vi "playback wrist.vi"(4 "Home":bool, 5 "Rewind":bool, 7 "Playback":bool, 8 "Taper Limit":dbl=1.0, 9 "Playback allow":bool=TRUE, 10 "Encoder Recording Data":cluster{dbl, u32}[](array[cluster])=[{0.0, 20}, {0.0, 41}, {0.0, 60}, {0.0, 80}, {0.0, 100}, {0.0, 120}, {0.0, 140}, {0.0, 160}, {0.0, 180}, {0.0, 200}, {0.0, 220}, {0.0, 245}, {0.0, 263}, {0.0, 284}, {0.0, 303}, {0.0, 325}, {0.0, 343}, {0.0, 364}, {0.0, 385}, {0.0, 406}, {0.0, 422}, {0.0, 442}, {0.0, 465}, {0.0, 486}, {0.0, 510}, {0.0, 527}, {0.0, 547}, {0.0, 567}, {0.0, 587}, {0.0, 606}, {0.0, 626}, {0.0, 649}, {0.0, 669}, {0.0, 689}, {0.0, 709}, {0.0, 730}, {0.0, 749}, {0.25, 769}, {0.75, 789}, {1.5, 809}, {2.75, 830}, {4.5, 849}, {7.25, 870}, {11.25, 891}, {16.25, 913}, {21.25, 931}, {28.5, 952}, {36.75, 974}, {45.75, 993}, {55.75, 1013}, {64.5, 1031}, {75.5, 1052}, {87.5, 1073}, {99.5, 1093}, {111.0, 1114}, {123.0, 1133}, {136.0, 1155}, {147.0, 1174}, {158.25, 1194}, {169.75, 1214}, {181.5, 1235}, {192.25, 1254}, {203.0, 1275}, {215.25, 1297}, {225.75, 1317}, {236.25, 1337}, {247.25, 1357}, {259.25, 1379}, {270.25, 1399}, {280.0, 1417}, {290.5, 1438}, {300.75, 1458}, {311.25, 1478}, {321.25, 1499}, {331.75, 1519}, {341.75, 1540}, {351.0, 1559}, {361.0, 1580}, {370.5, 1599}, {379.25, 1619}, {389.0, 1639}, {398.5, 1660}, {407.5, 1679}, {417.0, 1699}, {426.75, 1720}, {436.0, 1740}, {445.25, 1760}, {457.5, 1787}, {464.25, 1801}, {474.75, 1823}, {482.75, 1841}, {493.5, 1864}, {503.0, 1884}, {511.75, 1903}, {521.75, 1925}, {530.5, 1945}, {540.25, 1966}, {549.0, 1986}, {558.0, 2006}, {567.25, 2027}, {576.0, 2047}, {585.5, 2068}, {594.75, 2087}, {604.0, 2107}, {613.5, 2127}, {623.25, 2147}, {632.75, 2167}, {643.5, 2189}, {652.75, 2208}, {661.5, 2227}, {671.5, 2248}, {680.75, 2268}, {690.25, 2288}, {700.25, 2309}, {709.75, 2329}, {718.5, 2347}, {728.25, 2369}, {737.0, 2389}, {745.25, 2408}, {753.75, 2429}, {761.25, 2448}, {769.25, 2469}, {776.0, 2488}, {783.25, 2508}, {790.0, 2528}, {797.0, 2549}, {803.5, 2570}, {809.75, 2590}, {815.25, 2610}, {819.5, 2630}, {823.0, 2651}, {825.75, 2674}, {829.75, 2694}, {832.75, 2712}, {835.75, 2733}, {837.5, 2755}, {839.0, 2775}, {840.25, 2795}, {841.25, 2815}, {842.5, 2836}, {843.0, 2855}, {843.5, 2875}, {843.5, 2896}, {843.75, 2917}, {846.5, 2937}, {850.25, 2957}, {851.25, 2977}, {851.25, 2997}, {851.25, 3016}, {851.25, 3037}, {851.25, 3057}, {851.25, 3077}, {850.75, 3097}, {850.5, 3117}, {850.5, 3137}, {850.25, 3157}, {850.25, 3178}, {850.25, 3198}, {850.25, 3218}, {851.25, 3238}, {851.5, 3258}, {851.5, 3278}, {851.5, 3298}, {851.75, 3318}, {851.75, 3339}, {851.75, 3359}, {851.75, 3380}, {851.75, 3400}, {851.75, 3420}, {851.75, 3444}, {851.75, 3460}, {851.75, 3481}, {851.75, 3500}, {851.75, 3520}, {851.75, 3541}, {851.75, 3562}, {851.75, 3580}, {851.75, 3600}, {851.75, 3620}, {851.75, 3641}, {851.75, 3664}, {852.0, 3680}, {852.0, 3701}, {852.0, 3720}, {852.0, 3741}, {852.0, 3761}, {852.0, 3781}, {852.0, 3805}, {852.0, 3821}, {852.0, 3844}, {852.0, 3865}, {852.0, 3886}, {852.0, 3904}, {852.0, 3927}, {852.0, 3945}, {852.0, 3965}, {852.0, 3985}, {852.0, 4007}, {852.0, 4026}, {852.0, 4045}, {852.0, 4066}, {852.0, 4087}, {852.0, 4108}, {852.0, 4129}, {852.0, 4149}, {852.0, 4169}, {852.0, 4190}, {852.0, 4209}, {852.0, 4229}, {852.0, 4250}, {852.0, 4270}, {852.0, 4289}, {852.0, 4309}, {852.0, 4329}, {852.0, 4349}, {852.0, 4369}, {852.0, 4389}, {852.0, 4409}, {852.0, 4429}, {852.0, 4449}, {852.0, 4469}, {852.0, 4490}, {852.0, 4511}, {852.0, 4529}, {852.0, 4549}, {852.0, 4570}, {852.0, 4590}, {852.0, 4609}, {852.0, 4629}, {852.0, 4650}, {852.0, 4669}, {852.0, 4690}, {852.0, 4710}, {852.0, 4730}, {852.0, 4751}, {852.0, 4770}, {852.0, 4790}, {852.0, 4811}, {852.0, 4830}, {852.0, 4854}, {852.0, 4874}, {852.0, 4894}, {852.0, 4910}, {852.0, 4933}, {852.0, 4951}, {852.0, 4971}, {852.0, 4993}, {852.0, 5013}, {852.0, 5034}, {852.0, 5053}, {852.0, 5074}, {852.0, 5094}, {852.0, 5112}, {852.0, 5134}, {852.0, 5154}, {852.0, 5173}, {851.25, 5193}, {850.25, 5213}, {849.0, 5232}, {847.0, 5254}, {845.25, 5277}, {845.0, 5296}, {844.75, 5315}, {843.25, 5335}, {843.25, 5354}, {843.0, 5376}, {843.0, 5396}, {843.0, 5415}, {843.0, 5435}, {843.0, 5454}, {843.0, 5474}, {843.0, 5496}, {843.0, 5516}, {843.0, 5534}, {843.0, 5555}, {843.0, 5576}, {842.75, 5595}, {842.75, 5614}, {842.75, 5634}, {842.75, 5654}, {842.5, 5677}, {842.0, 5698}, {840.75, 5717}, {838.5, 5738}, {835.75, 5759}, {832.0, 5779}, {828.25, 5799}, {824.25, 5820}, {820.25, 5838}, {815.25, 5859}, {810.25, 5879}, {804.25, 5900}, {798.0, 5918}, {790.5, 5938}, {782.0, 5958}, {771.75, 5979}, {762.0, 5999}, {751.5, 6019}, {739.75, 6040}, {729.5, 6059}, {718.0, 6079}, {707.25, 6098}, {694.5, 6120}, {683.75, 6138}, {671.75, 6159}, {659.5, 6179}, {647.25, 6200}, {635.75, 6219}, {624.25, 6240}, {610.0, 6264}, {601.75, 6279}, {590.75, 6300}, {580.0, 6321}, {569.75, 6340}, {558.75, 6362}, {549.5, 6380}, {540.75, 6399}, {531.5, 6419}, {522.5, 6439}, {512.75, 6462}, {505.0, 6480}, {496.0, 6500}, {488.25, 6519}, {479.5, 6539}, {471.0, 6559}, {462.25, 6580}, {454.0, 6600}, {445.75, 6620}, {438.0, 6639}, {429.5, 6660}, {421.25, 6679}, {413.0, 6699}, {404.25, 6720}, {395.5, 6740}, {386.75, 6760}, {377.75, 6781}, {368.75, 6803}, {360.75, 6821}, {349.75, 6847}, {339.75, 6867}, {330.5, 6886}, {320.5, 6906}, {309.5, 6927}, {298.0, 6949}, {286.0, 6970}, {274.25, 6991}, {262.0, 7011}, {250.25, 7030}, {237.5, 7051}, {223.25, 7074}, {210.5, 7094}, {199.25, 7111}, {184.25, 7133}, {173.5, 7150}, {157.5, 7174}, {144.0, 7194}, {130.25, 7214}, {117.0, 7235}, {104.0, 7254}, {90.25, 7276}, {78.75, 7294}, {66.5, 7315}, {53.25, 7337}, {41.75, 7357}, {30.5, 7377}, {18.75, 7399}, {8.5, 7418}, {-0.75, 7438}, {-10.5, 7459}, {-19.75, 7479}, {-28.75, 7500}, {-36.5, 7521}, {-44.0, 7541}, {-51.5, 7562}, {-58.5, 7584}, {-63.75, 7603}, {-68.0, 7624}, {-70.75, 7643}, {-76.0, 7666}, {-80.25, 7686}, {-84.0, 7704}, {-87.5, 7724}, {-90.5, 7743}, {-93.75, 7766}, {-96.0, 7785}, {-98.25, 7807}, {-100.0, 7825}, {-101.5, 7845}, {-104.0, 7865}, {-108.0, 7885}, {-110.5, 7906}, {-111.25, 7927}, {-111.5, 7947}, {-112.25, 7967}, {-113.5, 7990}, {-115.0, 8006}, {-119.25, 8027}, {-124.0, 8047}, {-130.5, 8068}, {-136.75, 8086}, {-143.75, 8108}, {-150.5, 8128}, {-157.25, 8149}, {-162.5, 8167}, {-169.25, 8189}, {-175.5, 8208}, {-183.25, 8230}, {-191.25, 8251}, {-198.5, 8268}, {-209.5, 8293}, {-217.75, 8311}, {-227.5, 8333}, {-235.25, 8350}, {-246.5, 8374}, {-254.75, 8390}, {-264.5, 8410}, {-276.0, 8431}, {-287.0, 8451}, {-300.5, 8473}, {-313.25, 8493}, {-327.25, 8516}, {-340.0, 8535}, {-355.5, 8557}, {-369.75, 8578}, {-382.25, 8594}, {-398.25, 8615}, {-413.0, 8635}, {-430.25, 8657}, {-446.25, 8677}, {-462.5, 8697}, {-479.5, 8717}, {-495.25, 8736}, {-512.5, 8757}, {-530.0, 8777}, {-545.25, 8795}, {-564.0, 8818}, {-580.0, 8838}, {-595.25, 8857}, {-613.25, 8880}, {-626.0, 8896}, {-640.75, 8916}, {-657.0, 8938}, {-672.0, 8957}, {-688.5, 8980}, {-708.0, 9006}, {-717.5, 9019}, {-733.5, 9041}, {-744.5, 9057}, {-759.5, 9079}, {-777.75, 9106}, {-789.5, 9124}, {-799.25, 9140}, {-812.75, 9163}, {-823.25, 9178}, {-835.75, 9198}, {-848.75, 9220}, {-859.75, 9239}, {-872.25, 9260}, {-883.25, 9278}, {-895.0, 9299}, {-906.75, 9320}, {-917.0, 9338}, {-928.5, 9358}, {-939.75, 9378}, {-950.75, 9398}, {-961.5, 9418}, {-972.25, 9438}, {-983.5, 9458}, {-994.75, 9479}, {-1005.75, 9498}, {-1017.5, 9519}, {-1028.25, 9538}, {-1040.5, 9558}, {-1055.0, 9582}, {-1068.75, 9604}, {-1079.5, 9621}, {-1097.75, 9649}, {-1106.5, 9662}, {-1124.0, 9688}, {-1133.25, 9702}, {-1145.75, 9721}, {-1163.0, 9747}, {-1174.25, 9765}, {-1190.0, 9790}, {-1201.5, 9809}, {-1213.75, 9829}, {-1225.75, 9850}, {-1236.75, 9870}, {-1248.0, 9890}, {-1259.0, 9910}, {-1269.75, 9931}, {-1279.25, 9949}, {-1288.75, 9969}, {-1298.5, 9990}, {-1306.5, 10009}, {-1315.0, 10029}, {-1323.25, 10050}, {-1331.0, 10071}, {-1337.75, 10090}, {-1344.75, 10111}, {-1351.25, 10130}, {-1358.25, 10151}, {-1363.5, 10171}, {-1369.75, 10195}, {-1374.5, 10216}, {-1378.5, 10235}, {-1383.0, 10255}, {-1387.0, 10275}, {-1391.5, 10297}, {-1395.25, 10315}, {-1399.75, 10335}, {-1404.5, 10356}, {-1409.0, 10375}, {-1413.25, 10395}, {-1418.25, 10416}, {-1423.0, 10436}, {-1428.25, 10457}, {-1433.75, 10475}, {-1440.25, 10497}, {-1446.5, 10516}, {-1452.5, 10536}, {-1459.0, 10556}, {-1465.25, 10577}, {-1471.75, 10597}, {-1478.5, 10617}, {-1484.75, 10637}, {-1491.0, 10658}, {-1497.0, 10678}, {-1503.0, 10699}, {-1508.75, 10719}, {-1514.0, 10738}, {-1519.5, 10759}, {-1525.25, 10780}, {-1530.0, 10799}, {-1534.75, 10819}, {-1539.0, 10838}, {-1543.0, 10858}, {-1547.25, 10879}, {-1551.5, 10901}, {-1555.0, 10919}, {-1559.5, 10944}, {-1562.75, 10960}, {-1566.25, 10979}, {-1569.75, 11000}, {-1573.0, 11020}, {-1575.75, 11041}, {-1578.25, 11059}, {-1580.75, 11081}, {-1582.5, 11099}, {-1584.0, 11121}, {-1585.0, 11140}, {-1585.75, 11159}, {-1586.25, 11180}, {-1586.5, 11200}, {-1586.75, 11219}, {-1587.0, 11239}, {-1587.5, 11260}, {-1587.75, 11280}, {-1588.25, 11299}, {-1588.75, 11320}, {-1589.75, 11340}, {-1591.25, 11361}, {-1592.75, 11381}, {-1594.5, 11400}, {-1596.75, 11424}, {-1598.75, 11443}, {-1600.75, 11463}, {-1603.25, 11484}, {-1605.25, 11500}, {-1608.25, 11520}, {-1611.0, 11540}, {-1613.75, 11562}, {-1616.0, 11581}, {-1618.25, 11601}, {-1619.75, 11621}, {-1621.5, 11644}, {-1622.5, 11661}, {-1623.25, 11681}, {-1623.75, 11703}, {-1624.0, 11724}, {-1624.0, 11744}, {-1624.25, 11763}, {-1624.25, 11782}, {-1624.25, 11802}], 11 "Hardware In":T5={"Motor Selection"="Wrist", "EncoderDevRef"={"DevStatus"={"status"=FALSE, "code"=0, "source"=""}, "EncoderIndex"=enum."Enc 0", "CounterIndex"=enum."Invalid", "DistancePerCount"=1.0, "Decoding Type"=enum."4x"}}) -> (0 "Encoder Distance PB":dbl)   [LabVIEW 2017]
uses:
  <vilib>/Rock Robotics/WPI/Encoder/WPI_EncoderDevRef.ctl
  <vilib>/Rock Robotics/SystemInterfaces/Encoder/FPGA_EncoderIdx.ctl
  <vilib>/Rock Robotics/SystemInterfaces/Counter/FPGA_CounterCtrSystemIndex.ctl
  <vilib>/Rock Robotics/WPI/Encoder/WPI_EncoderType.ctl
  <vilib>/Rock Robotics/WPI/Utilities/WPI_GetSetVariantRefNum.vi
  <vilib>/addons/control/pid/pid.llb/PID (DBL).vi
  <vilib>/Rock Robotics/WPI/RobotDrive/WPI_RobotDriveArcadeDrive_Standard(NoSaturation).vi
  <vilib>/addons/control/pid/NI_PID_pid.lvlib
panel:
  out "Initial Encoder Position":dbl=-12.0
  out "Waveform Chart":cluster{dbl, dbl}(graph)={0.0, 40.5}
  in  "Playback PID gains":T6={"proportional gain (Kc)"=-0.01, "integral time (Ti, min)"=0.014, "derivative time (Td, min)"=0.0} {"derivative time (Td, min)" format="%.8f"; "integral time (Ti, min)" format="%.8f"; "proportional gain (Kc)" format="%.8f"}
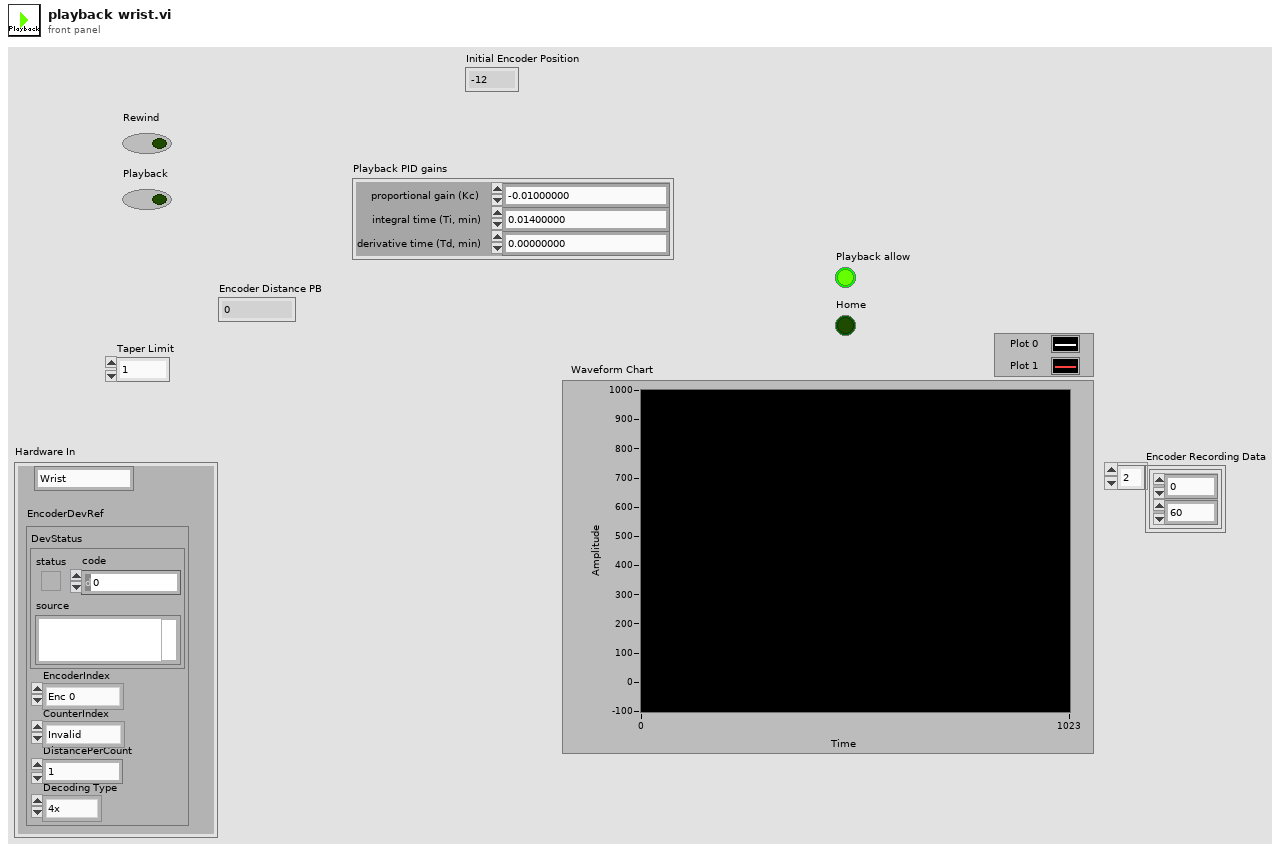
[diagram p1: front panel]
types:
  T1 = typedef "WPI_EncoderDevRef.ctl" = cluster{"DevStatus":errorcluster, "EncoderIndex":T2, "CounterIndex":T3, "DistancePerCount":dbl, "Decoding Type":T4}
  T2 = typedef "FPGA_EncoderIdx.ctl" = enum8{"Enc 0", "Enc 1", "Enc 2", "Enc 3", "Enc 4", "Enc 5", "Enc 6", "Enc 7", "Invalid"}
  T3 = typedef "FPGA_CounterCtrSystemIndex.ctl" = enum8{"Ctr 0", "Ctr 1", "Ctr 2", "Ctr 3", "Ctr 4", "Ctr 5", "Ctr 6", "Ctr 7", "Invalid"}
  T4 = typedef "WPI_EncoderType.ctl" = enum16{"1x", "2x", "4x"}
  T5 = cluster{"Motor Selection":string, "EncoderDevRef":T1}
  T6 = cluster{"proportional gain (Kc)":dbl, "integral time (Ti, min)":dbl, "derivative time (Td, min)":dbl}
  T7 = typedef "WPI_RobotDriveDevRef.ctl" = cluster{"DevStatus":errorcluster, "Motors[]":T8[], "Square Inputs":bool, "Max Output":dbl}
  T8 = typedef "WPI_MotorControlDeviceRef.ctl" = cluster{"DeviceStatus":errorcluster, "Type":T9, "PWM":cluster{"PWM Channel":T10, "DeadBand":T11}, "CAN":cluster{"Device Number":u8, "SetOutput VI Ref":variant, "GetOutput VI Ref":variant, "Enable VI Ref":variant, "Disable VI Ref":variant, "Data":variant}, "Invert":bool, "DIO PWM":cluster{"PWM \"Enable\" Channel":T10, "DIOChannel":T12, "PWM Rate":dbl}}
  T9 = typedef "WPI_MotorControlType.ctl" = enum16{"PWM", "CAN", "DIO PWM"}
  T10 = typedef "FPGA_DIOPWMChannel.ctl" = enum8{"PWM 0", "PWM 1", "PWM 2", "PWM 3", "PWM 4", "PWM 5", "PWM 6", "PWM 7", "PWM 8", "PWM 9", "PWM MXP 0", "PWM MXP 1", "PWM MXP 2", "PWM MXP 3", "PWM MXP 4", "PWM MXP 5", "PWM MXP 6", "PWM MXP 7", "PWM MXP 8", "PWM MXP 9", "Invalid"}
  T11 = typedef "WPI_PWMDeadband.ctl" = cluster{"Name":string, "maxPositivePwm":i32, "minPositivePwm":i32, "centerPwm":i32, "maxNegativePwm":i32, "minNegativePwm":i32, "angularRange":u16}
  T12 = typedef "FPGA_DIOChannel.ctl" = enum8{"DIO 0", "DIO 1", "DIO 2", "DIO 3", "DIO 4", "DIO 5", "DIO 6", "DIO 7", "DIO 8", "DIO 9", "DIO MXP 0", "DIO MXP 1", "DIO MXP 2", "DIO MXP 3", "DIO MXP 4", "DIO MXP 5", "DIO MXP 6", "DIO MXP 7", "DIO MXP 8", "DIO MXP 9", "DIO MXP 10", "DIO MXP 11", "DIO MXP 12", "DIO MXP 13", "DIO MXP 14", "DIO MXP 15", "SPI Port CS1", "SPI Port CS2", "SPI Port CS3", "SPI Port MISO", "SPI Port MOSI", "Invalid"}
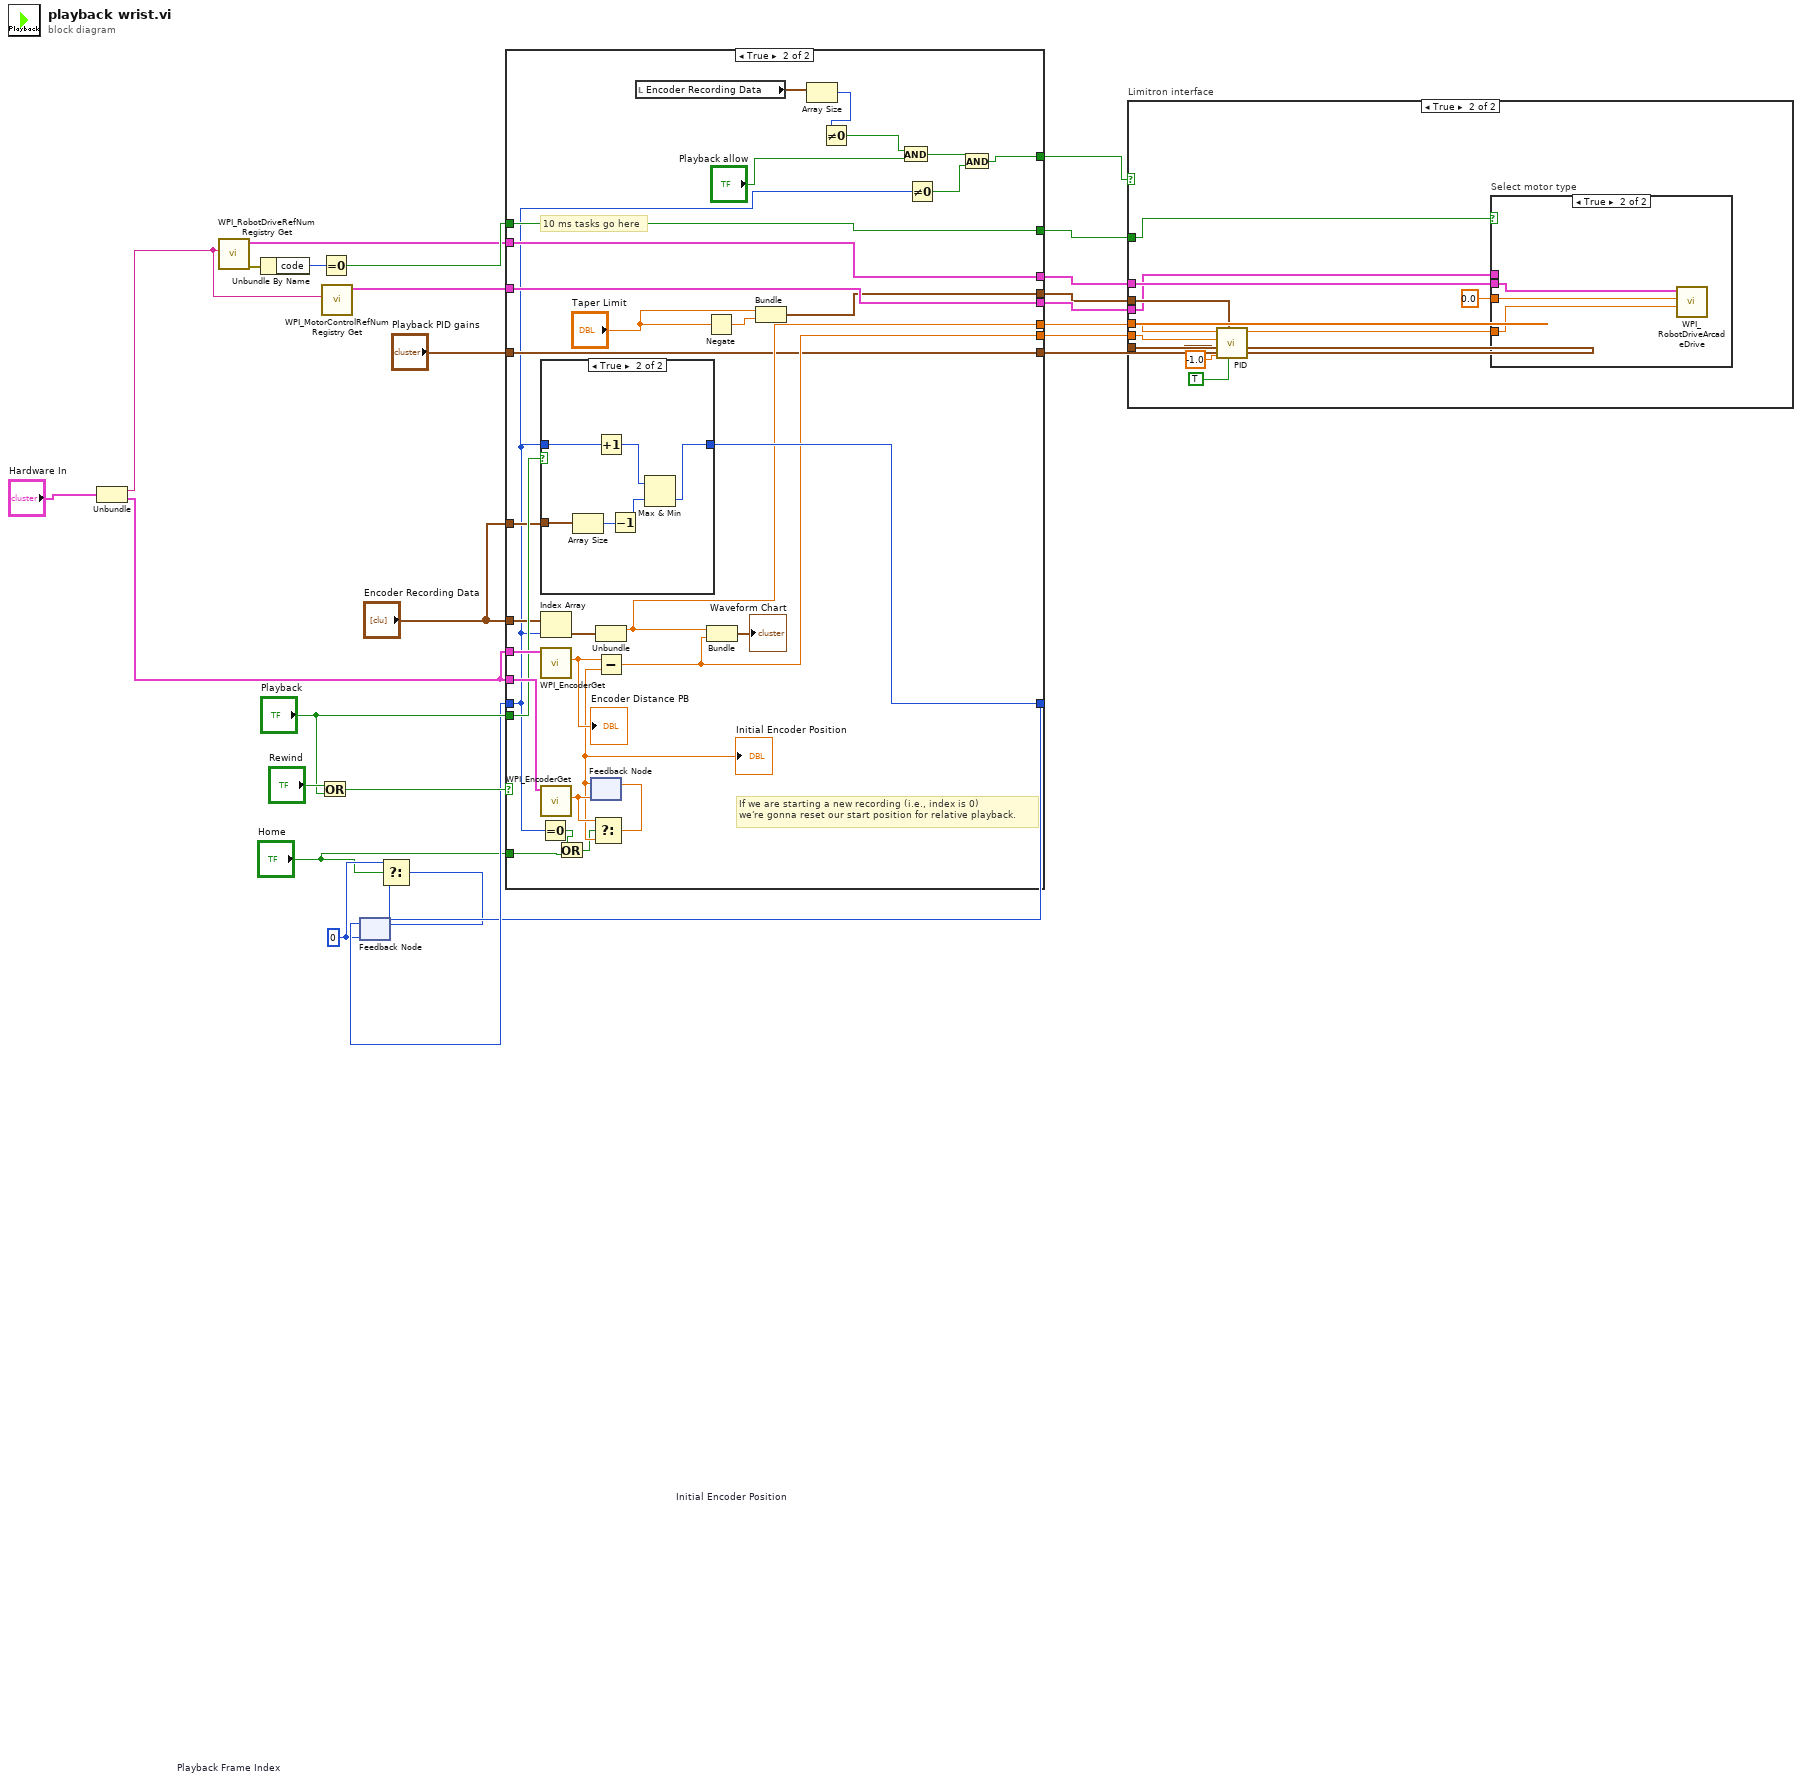
[diagram p0: block diagram]
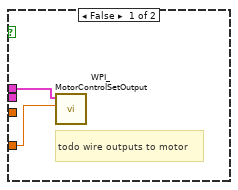
[diagram p3: hidden frame]
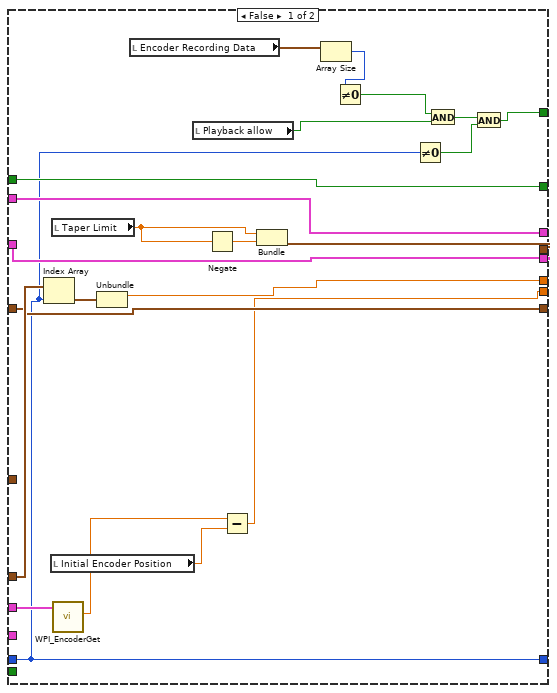
[diagram p4: hidden frame]
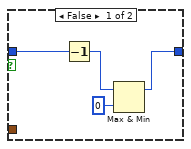
[diagram p5: hidden frame]
diagram:
  w15 = 0 ("index")
  n1 = Unbundle("Hardware In") -> ("Motor Selection"=w11:string, "EncoderDevRef"=w10:T1)
  n2 = call <vilib>:"WPI_RobotDriveRefNum Registry Get.vi"("refnum name"=w11) -> ("error out"=w25:errorcluster, "RobotDriveDevRef"=w23:T7)  [unwired: 1 in, 8 out]
  n3 = Unbundle By Name(w25) -> ("code"=w26:i32)
  n4 = Or(x="Rewind", y="Playback") -> (x .or. y?=w21:bool)
  n5 = Equal To 0?(x=w26) -> (x = 0?=w24:bool)
  n6 = call <vilib>:"WPI_MotorControlRefNum Registry Get.vi"("refnum name"=w11) -> ("MotorControlDevRef"=w19:T8)  [unwired: 9 in, 1 out]
  n7 = feedback #1 "Playback Frame Index"(w15) -> (w18:i32)
  n8 = case shown="True" w21 {
    tunnel: w10 -> [_ w80]
    tunnel: w10 -> [w34 w79]
    tunnel: w24 -> [w44 w67]
    tunnel: w23 -> [w43 w66]
    tunnel: "Playback" -> [_ w78]
    tunnel: w19 -> [w42 w65]
    tunnel: "Encoder Recording Data" -> [w48 w72]
    tunnel: w18 -> [w27 w52]
    tunnel: [w27 w71] -> w16
    tunnel: "Playback PID gains" -> [w40 w61]
    tunnel: "Encoder Recording Data" -> [_ w68]
    tunnel: [w44 w67] -> w9
    tunnel: [w43 w66] -> w8
    tunnel: [w42 w65] -> w7
    tunnel: [w41 w64] -> w6
    tunnel: [w31 w63] -> w5
    tunnel: [w39 w62] -> w4
    tunnel: [w40 w61] -> w3
    tunnel: [w29 w54] -> w2
    tunnel: "Home" -> [_ w49]
    frame False {
      n9 = Index Array(array=w48, index=w27) -> (element=w47:cluster{dbl, u32})
      n10 = local read "Initial Encoder Position"() -> (w32:dbl)
      n11 = local read "Taper Limit"() -> (w45:dbl)
      n12 = call <vilib>:"WPI_EncoderGet.vi"("EncoderDevRef"=w34) -> ("Distance"=w33:dbl)  [unwired: 5 in, 5 out]
      n13 = Unbundle(w47) -> (w41:dbl)  [unwired: 1 out]
      n14 = local read "Encoder Recording Data"() -> (w35:cluster{dbl, u32}[])
      n15 = local read "Playback allow"() -> (w36:bool)
      n16 = Negate(x=w45) -> (-x=w46:dbl)
      n17 = Subtract(x=w33, y=w32) -> (x-y=w31:dbl)
      n18 = Bundle("Taper Limit"=w45, w46) -> (w39:cluster{"Taper Limit":dbl, dbl})  [unwired: 1 in]
      n19 = Array Size(array=w35) -> (size(s)=w38:i32)
      n20 = Not Equal To 0?(x=w38) -> (x != 0?=w37:bool)
      n21 = Not Equal To 0?(x=w27) -> (x != 0?=w28:bool)
      n22 = And(x=w37, y=w36) -> (x .and. y?=w30:bool)
      n23 = And(x=w30, y=w28) -> (x .and. y?=w29:bool)
    }
    frame True {
      # "If we are starting a new recording (i.e., index is 0)\nwe're gonna reset our start position for relative playback."
      # "10 ms tasks go here"
      n24 = Equal To 0?(x=w52) -> (x = 0?=w51:bool)
      n25 = case shown="True" w78 {
        tunnel: [w81 w88] -> w71
        tunnel: w52 -> [w84 w90]
        tunnel: w68 -> [_ w87]
        frame False {
          n26 = Decrement(x=w84) -> (x-1=w82:i32)
          n27 = Max & Min(x=w82, y=0) -> (max(x,y)=w81:i32)  [unwired: 1 out]
        }
        frame True {
          n28 = Array Size(array=w87) -> (size(s)=w86:i32)
          n29 = Increment(x=w90) -> (x+1=w89:i32)
          n30 = Decrement(x=w86) -> (x-1=w85:i32)
          n31 = Max & Min(x=w89, y=w85) -> (min(x,y)=w88:i32)  [unwired: 1 out]
        }
      }
      n32 = Index Array(array=w72, index=w52) -> (element=w73:cluster{dbl, u32})
      n33 = call <vilib>:"WPI_EncoderGet.vi"("EncoderDevRef"=w79) -> ("Distance"=w77:dbl)  [unwired: 5 in, 5 out]
      "Encoder Distance PB" <- w77
      n34 = call <vilib>:"WPI_EncoderGet.vi"("EncoderDevRef"=w80) -> ("Distance"=w70:dbl)  [unwired: 5 in, 5 out]
      n35 = Or(x=w51, y=w49) -> (x .or. y?=w50:bool)
      n36 = feedback #2 "Initial Encoder Position"(w70) -> (w69:dbl)
      "Initial Encoder Position" <- w69
      n37 = Select(t=w70, s=w50, f=w69) -> (s? t:f=w56:dbl)
      n38 = feedback-in #2(w56) -> ()
      n39 = Unbundle(w73) -> (w64:dbl)  [unwired: 1 out]
      n40 = Subtract(x=w77, y=w69) -> (x-y=w63:dbl)
      n41 = local read "Encoder Recording Data"() -> (w59:cluster{dbl, u32}[])
      n42 = Negate(x="Taper Limit") -> (-x=w75:dbl)
      n43 = Bundle(w64, w63) -> (→"Waveform Chart":cluster{dbl, dbl})  [unwired: 1 in]
      n44 = Bundle("Taper Limit"="Taper Limit", w75) -> (w62:cluster{"Taper Limit":dbl, dbl})  [unwired: 1 in]
      n45 = Array Size(array=w59) -> (size(s)=w60:i32)
      n46 = Not Equal To 0?(x=w60) -> (x != 0?=w57:bool)
      n47 = And(x=w57, y="Playback allow") -> (x .and. y?=w55:bool)
      n48 = Not Equal To 0?(x=w52) -> (x != 0?=w53:bool)
      n49 = And(x=w55, y=w53) -> (x .and. y?=w54:bool)
    }
  }
  n50 = Select(t=w15, s="Home", f=w16) -> (s? t:f=w14:i32)
  n51 = feedback-in #1(w14) -> ()
  n52 = case "Limitron interface" shown="True" w2 {
    tunnel: w3 -> [_ w101]
    tunnel: w5 -> [_ w98]
    tunnel: w6 -> [_ w97]
    tunnel: w7 -> [_ w92]
    tunnel: w9 -> [_ w93]
    tunnel: w8 -> [_ w95]
    tunnel: w4 -> [_ w94]
    frame False {
    }
    frame True {
      n53 = call-poly <vilib>:"PID.vi"("reinitialize? (F)"=TRUE, "output range"=w94, "dt (s)"=-1.0, "PID gains"=w101, "process variable"=w98, "setpoint"=w97) -> ("output"=w96:dbl)  [unwired: 4 in, 1 out]
      n54 = case "Select motor type" shown="True" w93 {
        tunnel: 0.0 ("output") -> [_ w106]
        tunnel: w96 -> [w103 w105]
        tunnel: w95 -> [_ w104]
        tunnel: w92 -> [w102 _]
        frame False {
          # "todo wire outputs to motor"
          n55 = call <vilib>:"WPI_MotorControlSetOutput.vi"("Output"=w103, "MotorControlDevRef"=w102) -> ()  [unwired: 7 in, 3 out]
        }
        frame True {
          n56 = call-poly <vilib>:"WPI_RobotDriveArcadeDrive.vi"("Y axis value"=w105, "X axis value"=w106, "RobotDriveDevRef"=w104) -> ()  [unwired: 6 in, 3 out]
        }
      }
    }
  }
